vi "test Json Parser.vi"() -> ()   [LabVIEW 2018, in "Image Json Parser.lvclass"]
uses:
  Image Json Parser.lvclass
  Img Json Frames.ctl
  Img Json Meta.ctl
panel:
  out "data":cluster{"frames":T1[], "meta":T2}
  in  "text":string="{\"frames\": {\n\"rudolf-r-rudolf-r_0-0.png\":\n{\n  \"frame\": {\"x\":0,\"y\":0,\"w\":269,\"h\":269},\n  \"rotated\": false,\n  \"trimmed\": false,\n  \"spriteSourceSize\": {\"x\":0,\"y\":0,\"w\":269,\"h\":269},\n  \"sourceSize\": {\"w\":269,\"h\":269}\n},\n\"rudolf-r-rudolf-r_0-1.png\":\n{\n  \"frame\": {\"x\":270,\"y\":0,\"w\":269,\"h\":269},\n  \"rotated\": false,\n  \"trimmed\": false,\n  \"spriteSourceSize\": {\"x\":0,\"y\":0,\"w\":269,\"h\":269},\n  \"sourceSize\": {\"w\":269,\"h\":269}\n},\n\"rudolf-r-rudolf-r_0-2.png\":\n{\n  \"frame\": {\"x\":540,\"y\":0,\"w\":269,\"h\":269},\n  \"rotated\": false,\n  \"trimmed\": false,\n  \"spriteSourceSize\": {\"x\":0,\"y\":0,\"w\":269,\"h\":269},\n  \"sourceSize\": {\"w\":269,\"h\":269}\n},\n\"rudolf-r-rudolf-r_0-3.png\":\n{\n  \"frame\": {\"x\":810,\"y\":0,\"w\":269,\"h\":269},\n  \"rotated\": false,\n  \"trimmed\": false,\n  \"spriteSourceSize\": {\"x\":0,\"y\":0,\"w\":269,\"h\":269},\n  \"sourceSize\": {\"w\":269,\"h\":269}\n},\n\"rudolf-r-rudolf-r_0-4.png\":\n{\n  \"frame\": {\"x\":1080,\"y\":0,\"w\":269,\"h\":269},\n  \"rotated\": false,\n  \"trimmed\": false,\n  \"spriteSourceSize\": {\"x\":0,\"y\":0,\"w\":269,\"h\":269},\n  \"sourceSize\": {\"w\":269,\"h\":269}\n},\n\"rudolf-r-rudolf-r_0-5.png\":\n{\n  \"frame\": {\"x\":1350,\"y\":0,\"w\":269,\"h\":269},\n  \"rotated\": false,\n  \"trimmed\": false,\n  \"spriteSourceSize\": {\"x\":0,\"y\":0,\"w\":269,\"h\":269},\n  \"sourceSize\": {\"w\":269,\"h\":269}\n},\n\"rudolf-r-rudolf-r_0-6.png\":\n{\n  \"frame\": {\"x\":1620,\"y\":0,\"w\":269,\"h\":269},\n  \"rotated\": false,\n  \"trimmed\": false,\n  \"spriteSourceSize\": {\"x\":0,\"y\":0,\"w\":269,\"h\":269},\n  \"sourceSize\": {\"w\":269,\"h\":269}\n},\n\"rudolf-r-rudolf-r_0-7.png\":\n{\n  \"frame\": {\"x\":1890,\"y\":0,\"w\":269,\"h\":269},\n  \"rotated\": false,\n  \"trimmed\": false,\n  \"spriteSourceSize\": {\"x\":0,\"y\":0,\"w\":269,\"h\":269},\n  \"sourceSize\": {\"w\":269,\"h\":269}\n},\n\"rudolf-r-rudolf-r_0-8.png\":\n{\n  \"frame\": {\"x\":2160,\"y\":0,\"w\":269,\"h\":269},\n  \"rotated\": false,\n  \"trimmed\": false,\n  \"spriteSourceSize\": {\"x\":0,\"y\":0,\"w\":269,\"h\":269},\n  \"sourceSize\": {\"w\":269,\"h\":269}\n},\n\"rudolf-r-rudolf-r_0-9.png\":\n{\n  \"frame\": {\"x\":2430,\"y\":0,\"w\":269,\"h\":269},\n  \"rotated\": false,\n  \"trimmed\": false,\n  \"spriteSourceSize\": {\"x\":0,\"y\":0,\"w\":269,\"h\":269},\n  \"sourceSize\": {\"w\":269,\"h\":269}\n},\n\"rudolf-r-rudolf-r_0-10.png\":\n{\n  \"frame\": {\"x\":0,\"y\":270,\"w\":269,\"h\":269},\n  \"rotated\": false,\n  \"trimmed\": false,\n  \"spriteSourceSize\": {\"x\":0,\"y\":0,\"w\":269,\"h\":269},\n  \"sourceSize\": {\"w\":269,\"h\":269}\n},\n\"rudolf-r-rudolf-r_0-11.png\":\n{\n  \"frame\": {\"x\":270,\"y\":270,\"w\":269,\"h\":269},\n  \"rotated\": false,\n  \"trimmed\": false,\n  \"spriteSourceSize\": {\"x\":0,\"y\":0,\"w\":269,\"h\":269},\n  \"sourceSize\": {\"w\":269,\"h\":269}\n},\n\"rudolf-r-rudolf-r_0-12.png\":\n{\n  \"frame\": {\"x\":540,\"y\":270,\"w\":269,\"h\":269},\n  \"rotated\": false,\n  \"trimmed\": false,\n  \"spriteSourceSize\": {\"x\":0,\"y\":0,\"w\":269,\"h\":269},\n  \"sourceSize\": {\"w\":269,\"h\":269}\n},\n\"rudolf-r-rudolf-r_0-13.png\":\n{\n  \"frame\": {\"x\":810,\"y\":270,\"w\":269,\"h\":269},\n  \"rotated\": false,\n  \"trimmed\": false,\n  \"spriteSourceSize\": {\"x\":0,\"y\":0,\"w\":269,\"h\":269},\n  \"sourceSize\": {\"w\":269,\"h\":269}\n},\n\"rudolf-r-rudolf-r_0-14.png\":\n{\n  \"frame\": {\"x\":1080,\"y\":270,\"w\":269,\"h\":269},\n  \"rotated\": false,\n  \"trimmed\": false,\n  \"spriteSourceSize\": {\"x\":0,\"y\":0,\"w\":269,\"h\":269},\n  \"sourceSize\": {\"w\":269,\"h\":269}\n},\n\"rudolf-r-rudolf-r_0-15.png\":\n{\n  \"frame\": {\"x\":1350,\"y\":270,\"w\":269,\"h\":269},\n  \"rotated\": false,\n  \"trimmed\": false,\n  \"spriteSourceSize\": {\"x\":0,\"y\":0,\"w\":269,\"h\":269},\n  \"sourceSize\": {\"w\":269,\"h\":269}\n},\n\"rudolf-r-rudolf-r_0-16.png\":\n{\n  \"frame\": {\"x\":1620,\"y\":270,\"w\":269,\"h\":269},\n  \"rotated\": false,\n  \"trimmed\": false,\n  \"spriteSourceSize\": {\"x\":0,\"y\":0,\"w\":269,\"h\":269},\n  \"sourceSize\": {\"w\":269,\"h\":269}\n},\n\"rudolf-r-rudolf-r_0-17.png\":\n{\n  \"frame\": {\"x\":1890,\"y\":270,\"w\":269,\"h\":269},\n  \"rotated\": false,\n  \"trimmed\": false,\n  \"spriteSourceSize\": {\"x\":0,\"y\":0,\"w\":269,\"h\":269},\n  \"sourceSize\": {\"w\":269,\"h\":269}\n},\n\"rudolf-r-rudolf-r_0-18.png\":\n{\n  \"frame\": {\"x\":2160,\"y\":270,\"w\":269,\"h\":269},\n  \"rotated\": false,\n  \"trimmed\": false,\n  \"spriteSourceSize\": {\"x\":0,\"y\":0,\"w\":269,\"h\":269},\n  \"sourceSize\": {\"w\":269,\"h\":269}\n},\n\"rudolf-r-rudolf-r_0-19.png\":\n{\n  \"frame\": {\"x\":2430,\"y\":270,\"w\":269,\"h\":269},\n  \"rotated\": false,\n  \"trimmed\": false,\n  \"spriteSourceSize\": {\"x\":0,\"y\":0,\"w\":269,\"h\":269},\n  \"sourceSize\": {\"w\":269,\"h\":269}\n},\n\"rudolf-r-rudolf-r_0-20.png\":\n{\n  \"frame\": {\"x\":0,\"y\":540,\"w\":269,\"h\":269},\n  \"rotated\": false,\n  \"trimmed\": false,\n  \"spriteSourceSize\": {\"x\":0,\"y\":0,\"w\":269,\"h\":269},\n  \"sourceSize\": {\"w\":269,\"h\":269}\n},\n\"rudolf-r-rudolf-r_0-21.png\":\n{\n  \"frame\": {\"x\":270,\"y\":540,\"w\":269,\"h\":269},\n  \"rotated\": false,\n  \"trimmed\": false,\n  \"spriteSourceSize\": {\"x\":0,\"y\":0,\"w\":269,\"h\":269},\n  \"sourceSize\": {\"w\":269,\"h\":269}\n},\n\"rudolf-r-rudolf-r_0-22.png\":\n{\n  \"frame\": {\"x\":540,\"y\":540,\"w\":269,\"h\":269},\n  \"rotated\": false,\n  \"trimmed\": false,\n  \"spriteSourceSize\": {\"x\":0,\"y\":0,\"w\":269,\"h\":269},\n  \"sourceSize\": {\"w\":269,\"h\":269}\n},\n\"rudolf-r-rudolf-r_0-23.png\":\n{\n  \"frame\": {\"x\":810,\"y\":540,\"w\":269,\"h\":269},\n  \"rotated\": false,\n  \"trimmed\": false,\n  \"spriteSourceSize\": {\"x\":0,\"y\":0,\"w\":269,\"h\":269},\n  \"sourceSize\": {\"w\":269,\"h\":269}\n},\n\"rudolf-r-rudolf-r_0-24.png\":\n{\n  \"frame\": {\"x\":1080,\"y\":540,\"w\":269,\"h\":269},\n  \"rotated\": false,\n  \"trimmed\": false,\n  \"spriteSourceSize\": {\"x\":0,\"y\":0,\"w\":269,\"h\":269},\n  \"sourceSize\": {\"w\":269,\"h\":269}\n},\n\"rudolf-r-rudolf-r_0-25.png\":\n{\n  \"frame\": {\"x\":1350,\"y\":540,\"w\":269,\"h\":269},\n  \"rotated\": false,\n  \"trimmed\": false,\n  \"spriteSourceSize\": {\"x\":0,\"y\":0,\"w\":269,\"h\":269},\n  \"sourceSize\": {\"w\":269,\"h\":269}\n},\n\"rudolf-r-rudolf-r_0-26.png\":\n{\n  \"frame\": {\"x\":1620,\"y\":540,\"w\":269,\"h\":269},\n  \"rotated\": false,\n  \"trimmed\": false,\n  \"spriteSourceSize\": {\"x\":0,\"y\":0,\"w\":269,\"h\":269},\n  \"sourceSize\": {\"w\":269,\"h\":269}\n},\n\"rudolf-r-rudolf-r_0-27.png\":\n{\n  \"frame\": {\"x\":1890,\"y\":540,\"w\":269,\"h\":269},\n  \"rotated\": false,\n  \"trimmed\": false,\n  \"spriteSourceSize\": {\"x\":0,\"y\":0,\"w\":269,\"h\":269},\n  \"sourceSize\": {\"w\":269,\"h\":269}\n},\n\"rudolf-r-rudolf-r_0-28.png\":\n{\n  \"frame\": {\"x\":2160,\"y\":540,\"w\":269,\"h\":269},\n  \"rotated\": false,\n  \"trimmed\": false,\n  \"spriteSourceSize\": {\"x\":0,\"y\":0,\"w\":269,\"h\":269},\n  \"sourceSize\": {\"w\":269,\"h\":269}\n},\n\"rudolf-r-rudolf-r_0-29.png\":\n{\n  \"frame\": {\"x\":2430,\"y\":540,\"w\":269,\"h\":269},\n  \"rotated\": false,\n  \"trimmed\": false,\n  \"spriteSourceSize\": {\"x\":0,\"y\":0,\"w\":269,\"h\":269},\n  \"sourceSize\": {\"w\":269,\"h\":269}\n},\n\"rudolf-r-rudolf-r_0-30.png\":\n{\n  \"frame\": {\"x\":0,\"y\":810,\"w\":269,\"h\":269},\n  \"rotated\": false,\n  \"trimmed\": false,\n  \"spriteSourceSize\": {\"x\":0,\"y\":0,\"w\":269,\"h\":269},\n  \"sourceSize\": {\"w\":269,\"h\":269}\n},\n\"rudolf-r-rudolf-r_0-31.png\":\n{\n  \"frame\": {\"x\":270,\"y\":810,\"w\":269,\"h\":269},\n  \"rotated\": false,\n  \"trimmed\": false,\n  \"spriteSourceSize\": {\"x\":0,\"y\":0,\"w\":269,\"h\":269},\n  \"sourceSize\": {\"w\":269,\"h\":269}\n},\n\"rudolf-r-rudolf-r_0-32.png\":\n{\n  \"frame\": {\"x\":540,\"y\":810,\"w\":269,\"h\":269},\n  \"rotated\": false,\n  \"trimmed\": false,\n  \"spriteSourceSize\": {\"x\":0,\"y\":0,\"w\":269,\"h\":269},\n  \"sourceSize\": {\"w\":269,\"h\":269}\n},\n\"rudolf-r-rudolf-r_0-33.png\":\n{\n  \"frame\": {\"x\":810,\"y\":810,\"w\":269,\"h\":269},\n  \"rotated\": false,\n  \"trimmed\": false,\n  \"spriteSourceSize\": {\"x\":0,\"y\":0,\"w\":269,\"h\":269},\n  \"sourceSize\": {\"w\":269,\"h\":269}\n},\n\"rudolf-r-rudolf-r_0-34.png\":\n{\n  \"frame\": {\"x\":1080,\"y\":810,\"w\":269,\"h\":269},\n  \"rotated\": false,\n  \"trimmed\": false,\n  \"spriteSourceSize\": {\"x\":0,\"y\":0,\"w\":269,\"h\":269},\n  \"sourceSize\": {\"w\":269,\"h\":269}\n},\n\"rudolf-r-rudolf-r_0-35.png\":\n{\n  \"frame\": {\"x\":1350,\"y\":810,\"w\":269,\"h\":269},\n  \"rotated\": false,\n  \"trimmed\": false,\n  \"spriteSourceSize\": {\"x\":0,\"y\":0,\"w\":269,\"h\":269},\n  \"sourceSize\": {\"w\":269,\"h\":269}\n},\n\"rudolf-r-rudolf-r_0-36.png\":\n{\n  \"frame\": {\"x\":1620,\"y\":810,\"w\":269,\"h\":269},\n  \"rotated\": false,\n  \"trimmed\": false,\n  \"spriteSourceSize\": {\"x\":0,\"y\":0,\"w\":269,\"h\":269},\n  \"sourceSize\": {\"w\":269,\"h\":269}\n},\n\"rudolf-r-rudolf-r_0-37.png\":\n{\n  \"frame\": {\"x\":1890,\"y\":810,\"w\":269,\"h\":269},\n  \"rotated\": false,\n  \"trimmed\": false,\n  \"spriteSourceSize\": {\"x\":0,\"y\":0,\"w\":269,\"h\":269},\n  \"sourceSize\": {\"w\":269,\"h\":269}\n},\n\"rudolf-r-rudolf-r_0-38.png\":\n{\n  \"frame\": {\"x\":2160,\"y\":810,\"w\":269,\"h\":269},\n  \"rotated\": false,\n  \"trimmed\": false,\n  \"spriteSourceSize\": {\"x\":0,\"y\":0,\"w\":269,\"h\":269},\n  \"sourceSize\": {\"w\":269,\"h\":269}\n},\n\"rudolf-r-rudolf-r_0-39.png\":\n{\n  \"frame\": {\"x\":2430,\"y\":810,\"w\":269,\"h\":269},\n  \"rotated\": false,\n  \"trimmed\": false,\n  \"spriteSourceSize\": {\"x\":0,\"y\":0,\"w\":269,\"h\":269},\n  \"sourceSize\": {\"w\":269,\"h\":269}\n},\n\"rudolf-r-rudolf-r_0-40.png\":\n{\n  \"frame\": {\"x\":0,\"y\":1080,\"w\":269,\"h\":269},\n  \"rotated\": false,\n  \"trimmed\": false,\n  \"spriteSourceSize\": {\"x\":0,\"y\":0,\"w\":269,\"h\":269},\n  \"sourceSize\": {\"w\":269,\"h\":269}\n},\n\"rudolf-r-rudolf-r_0-41.png\":\n{\n  \"frame\": {\"x\":270,\"y\":1080,\"w\":269,\"h\":269},\n  \"rotated\": false,\n  \"trimmed\": false,\n  \"spriteSourceSize\": {\"x\":0,\"y\":0,\"w\":269,\"h\":269},\n  \"sourceSize\": {\"w\":269,\"h\":269}\n},\n\"rudolf-r-rudolf-r_0-42.png\":\n{\n  \"frame\": {\"x\":540,\"y\":1080,\"w\":269,\"h\":269},\n  \"rotated\": false,\n  \"trimmed\": false,\n  \"spriteSourceSize\": {\"x\":0,\"y\":0,\"w\":269,\"h\":269},\n  \"sourceSize\": {\"w\":269,\"h\":269}\n},\n\"rudolf-r-rudolf-r_0-43.png\":\n{\n  \"frame\": {\"x\":810,\"y\":1080,\"w\":269,\"h\":269},\n  \"rotated\": false,\n  \"trimmed\": false,\n  \"spriteSourceSize\": {\"x\":0,\"y\":0,\"w\":269,\"h\":269},\n  \"sourceSize\": {\"w\":269,\"h\":269}\n},\n\"rudolf-r-rudolf-r_0-44.png\":\n{\n  \"frame\": {\"x\":1080,\"y\":1080,\"w\":269,\"h\":269},\n  \"rotated\": false,\n  \"trimmed\": false,\n  \"spriteSourceSize\": {\"x\":0,\"y\":0,\"w\":269,\"h\":269},\n  \"sourceSize\": {\"w\":269,\"h\":269}\n},\n\"rudolf-r-rudolf-r_0-45.png\":\n{\n  \"frame\": {\"x\":1350,\"y\":1080,\"w\":269,\"h\":269},\n  \"rotated\": false,\n  \"trimmed\": false,\n  \"spriteSourceSize\": {\"x\":0,\"y\":0,\"w\":269,\"h\":269},\n  \"sourceSize\": {\"w\":269,\"h\":269}\n},\n\"rudolf-r-rudolf-r_0-46.png\":\n{\n  \"frame\": {\"x\":1620,\"y\":1080,\"w\":269,\"h\":269},\n  \"rotated\": false,\n  \"trimmed\": false,\n  \"spriteSourceSize\": {\"x\":0,\"y\":0,\"w\":269,\"h\":269},\n  \"sourceSize\": {\"w\":269,\"h\":269}\n},\n\"rudolf-r-rudolf-r_0-47.png\":\n{\n  \"frame\": {\"x\":1890,\"y\":1080,\"w\":269,\"h\":269},\n  \"rotated\": false,\n  \"trimmed\": false,\n  \"spriteSourceSize\": {\"x\":0,\"y\":0,\"w\":269,\"h\":269},\n  \"sourceSize\": {\"w\":269,\"h\":269}\n},\n\"rudolf-r-rudolf-r_0-48.png\":\n{\n  \"frame\": {\"x\":2160,\"y\":1080,\"w\":269,\"h\":269},\n  \"rotated\": false,\n  \"trimmed\": false,\n  \"spriteSourceSize\": {\"x\":0,\"y\":0,\"w\":269,\"h\":269},\n  \"sourceSize\": {\"w\":269,\"h\":269}\n},\n\"rudolf-r-rudolf-r_0-49.png\":\n{\n  \"frame\": {\"x\":2430,\"y\":1080,\"w\":269,\"h\":269},\n  \"rotated\": false,\n  \"trimmed\": false,\n  \"spriteSourceSize\": {\"x\":0,\"y\":0,\"w\":269,\"h\":269},\n  \"sourceSize\": {\"w\":269,\"h\":269}\n},\n\"rudolf-r-rudolf-r_0-50.png\":\n{\n  \"frame\": {\"x\":0,\"y\":1350,\"w\":269,\"h\":269},\n  \"rotated\": false,\n  \"trimmed\": false,\n  \"spriteSourceSize\": {\"x\":0,\"y\":0,\"w\":269,\"h\":269},\n  \"sourceSize\": {\"w\":269,\"h\":269}\n},\n\"rudolf-r-rudolf-r_0-51.png\":\n{\n  \"frame\": {\"x\":270,\"y\":1350,\"w\":269,\"h\":269},\n  \"rotated\": false,\n  \"trimmed\": false,\n  \"spriteSourceSize\": {\"x\":0,\"y\":0,\"w\":269,\"h\":269},\n  \"sourceSize\": {\"w\":269,\"h\":269}\n},\n\"rudolf-r-rudolf-r_0-52.png\":\n{\n  \"frame\": {\"x\":540,\"y\":1350,\"w\":269,\"h\":269},\n  \"rotated\": false,\n  \"trimmed\": false,\n  \"spriteSourceSize\": {\"x\":0,\"y\":0,\"w\":269,\"h\":269},\n  \"sourceSize\": {\"w\":269,\"h\":269}\n},\n\"rudolf-r-rudolf-r_0-53.png\":\n{\n  \"frame\": {\"x\":810,\"y\":1350,\"w\":269,\"h\":269},\n  \"rotated\": false,\n  \"trimmed\": false,\n  \"spriteSourceSize\": {\"x\":0,\"y\":0,\"w\":269,\"h\":269},\n  \"sourceSize\": {\"w\":269,\"h\":269}\n},\n\"rudolf-r-rudolf-r_0-54.png\":\n{\n  \"frame\": {\"x\":1080,\"y\":1350,\"w\":269,\"h\":269},\n  \"rotated\": false,\n  \"trimmed\": false,\n  \"spriteSourceSize\": {\"x\":0,\"y\":0,\"w\":269,\"h\":269},\n  \"sourceSize\": {\"w\":269,\"h\":269}\n},\n\"rudolf-r-rudolf-r_0-55.png\":\n{\n  \"frame\": {\"x\":1350,\"y\":1350,\"w\":269,\"h\":269},\n  \"rotated\": false,\n  \"trimmed\": false,\n  \"spriteSourceSize\": {\"x\":0,\"y\":0,\"w\":269,\"h\":269},\n  \"sourceSize\": {\"w\":269,\"h\":269}\n},\n\"rudolf-r-rudolf-r_0-56.png\":\n{\n  \"frame\": {\"x\":1620,\"y\":1350,\"w\":269,\"h\":269},\n  \"rotated\": false,\n  \"trimmed\": false,\n  \"spriteSourceSize\": {\"x\":0,\"y\":0,\"w\":269,\"h\":269},\n  \"sourceSize\": {\"w\":269,\"h\":269}\n},\n\"rudolf-r-rudolf-r_0-57.png\":\n{\n  \"frame\": {\"x\":1890,\"y\":1350,\"w\":269,\"h\":269},\n  \"rotated\": false,\n  \"trimmed\": false,\n  \"spriteSourceSize\": {\"x\":0,\"y\":0,\"w\":269,\"h\":269},\n  \"sourceSize\": {\"w\":269,\"h\":269}\n},\n\"rudolf-r-rudolf-r_0-58.png\":\n{\n  \"frame\": {\"x\":2160,\"y\":1350,\"w\":269,\"h\":269},\n  \"rotated\": false,\n  \"trimmed\": false,\n  \"spriteSourceSize\": {\"x\":0,\"y\":0,\"w\":269,\"h\":269},\n  \"sourceSize\": {\"w\":269,\"h\":269}\n},\n\"rudolf-r-rudolf-r_0-59.png\":\n{\n  \"frame\": {\"x\":2430,\"y\":1350,\"w\":269,\"h\":269},\n  \"rotated\": false,\n  \"trimmed\": false,\n  \"spriteSourceSize\": {\"x\":0,\"y\":0,\"w\":269,\"h\":269},\n  \"sourceSize\": {\"w\":269,\"h\":269}\n},\n\"rudolf-r-rudolf-r_0-60.png\":\n{\n  \"frame\": {\"x\":0,\"y\":1620,\"w\":269,\"h\":269},\n  \"rotated\": false,\n  \"trimmed\": false,\n  \"spriteSourceSize\": {\"x\":0,\"y\":0,\"w\":269,\"h\":269},\n  \"sourceSize\": {\"w\":269,\"h\":269}\n},\n\"rudolf-r-rudolf-r_0-61.png\":\n{\n  \"frame\": {\"x\":270,\"y\":1620,\"w\":269,\"h\":269},\n  \"rotated\": false,\n  \"trimmed\": false,\n  \"spriteSourceSize\": {\"x\":0,\"y\":0,\"w\":269,\"h\":269},\n  \"sourceSize\": {\"w\":269,\"h\":269}\n},\n\"rudolf-r-rudolf-r_0-62.png\":\n{\n  \"frame\": {\"x\":540,\"y\":1620,\"w\":269,\"h\":269},\n  \"rotated\": false,\n  \"trimmed\": false,\n  \"spriteSourceSize\": {\"x\":0,\"y\":0,\"w\":269,\"h\":269},\n  \"sourceSize\": {\"w\":269,\"h\":269}\n},\n\"rudolf-r-rudolf-r_0-63.png\":\n{\n  \"frame\": {\"x\":810,\"y\":1620,\"w\":269,\"h\":269},\n  \"rotated\": false,\n  \"trimmed\": false,\n  \"spriteSourceSize\": {\"x\":0,\"y\":0,\"w\":269,\"h\":269},\n  \"sourceSize\": {\"w\":269,\"h\":269}\n},\n\"rudolf-r-rudolf-r_0-64.png\":\n{\n  \"frame\": {\"x\":1080,\"y\":1620,\"w\":269,\"h\":269},\n  \"rotated\": false,\n  \"trimmed\": false,\n  \"spriteSourceSize\": {\"x\":0,\"y\":0,\"w\":269,\"h\":269},\n  \"sourceSize\": {\"w\":269,\"h\":269}\n},\n\"rudolf-r-rudolf-r_0-65.png\":\n{\n  \"frame\": {\"x\":1350,\"y\":1620,\"w\":269,\"h\":269},\n  \"rotated\": false,\n  \"trimmed\": false,\n  \"spriteSourceSize\": {\"x\":0,\"y\":0,\"w\":269,\"h\":269},\n  \"sourceSize\": {\"w\":269,\"h\":269}\n},\n\"rudolf-r-rudolf-r_0-66.png\":\n{\n  \"frame\": {\"x\":1620,\"y\":1620,\"w\":269,\"h\":269},\n  \"rotated\": false,\n  \"trimmed\": false,\n  \"spriteSourceSize\": {\"x\":0,\"y\":0,\"w\":269,\"h\":269},\n  \"sourceSize\": {\"w\":269,\"h\":269}\n},\n\"rudolf-r-rudolf-r_0-67.png\":\n{\n  \"frame\": {\"x\":1890,\"y\":1620,\"w\":269,\"h\":269},\n  \"rotated\": false,\n  \"trimmed\": false,\n  \"spriteSourceSize\": {\"x\":0,\"y\":0,\"w\":269,\"h\":269},\n  \"sourceSize\": {\"w\":269,\"h\":269}\n},\n\"rudolf-r-rudolf-r_0-68.png\":\n{\n  \"frame\": {\"x\":2160,\"y\":1620,\"w\":269,\"h\":269},\n  \"rotated\": false,\n  \"trimmed\": false,\n  \"spriteSourceSize\": {\"x\":0,\"y\":0,\"w\":269,\"h\":269},\n  \"sourceSize\": {\"w\":269,\"h\":269}\n},\n\"rudolf-r-rudolf-r_0-69.png\":\n{\n  \"frame\": {\"x\":2430,\"y\":1620,\"w\":269,\"h\":269},\n  \"rotated\": false,\n  \"trimmed\": false,\n  \"spriteSourceSize\": {\"x\":0,\"y\":0,\"w\":269,\"h\":269},\n  \"sourceSize\": {\"w\":269,\"h\":269}\n}},\n\"meta\": {\n  \"app\": \"LF2 remaster\",\n  \"version\": \".1\",\n  \"image\": \"rudolf-r_0.png\",\n  \"format\": \"RGBA8888\",\n  \"size\": {\"w\":1,\"h\":1},\n  \"scale\": \"1\"\n}\n}\n"
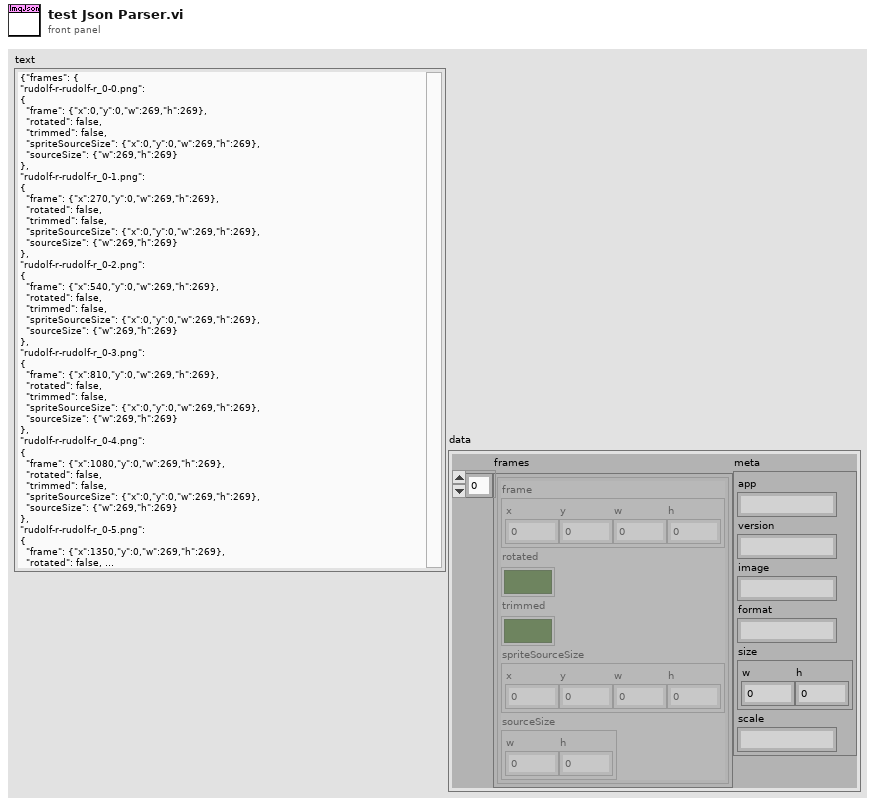
[diagram p1: front panel]
types:
  T1 = typedef "Image Json Parser.lvclass/Img Json Frames.ctl" = cluster{"frame":cluster{"x":i32, "y":i32, "w":i32, "h":i32}, "rotated":bool, "trimmed":bool, "spriteSourceSize":cluster{"x":i32, "y":i32, "w":i32, "h":i32}, "sourceSize":cluster{"w":i32, "h":i32}}
  T2 = typedef "Image Json Parser.lvclass/Img Json Meta.ctl" = cluster{"app":string, "version":string, "image":string, "format":string, "size":cluster{"w":i32, "h":i32}, "scale":string}
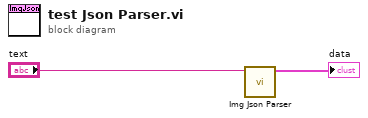
[diagram p0: block diagram]
diagram:
  n1 = call "Img Json Parser.vi"("Json string"="text") -> ("data"=→"data":cluster{"frames":T1[], "meta":T2})  [unwired: 8 in, 2 out]
